vi "Copy Class.vi"(5 "Parent Class Path":path, 7 "Template Path":path, 8 "error in (no error)":errorcluster, 9 "Class Name":string, 10 "Destination Directory":path, 11 "AppInst":refnum<vi>) -> (0 "error out":errorcluster, 2 "New Class Path":path)   [LabVIEW 2020, in "Message Maker.lvlib"]
uses:
  Message Maker.lvlib
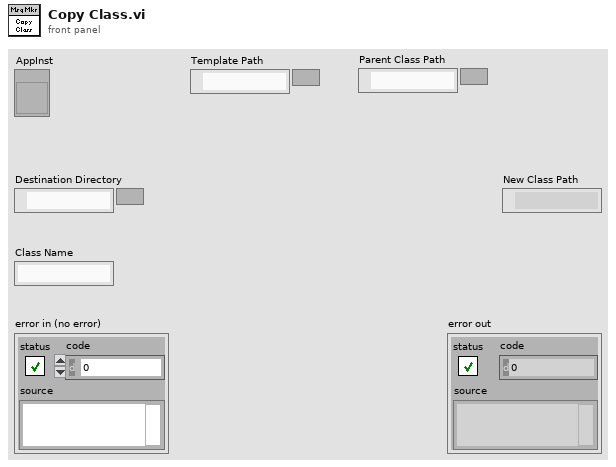
[diagram p1: front panel]
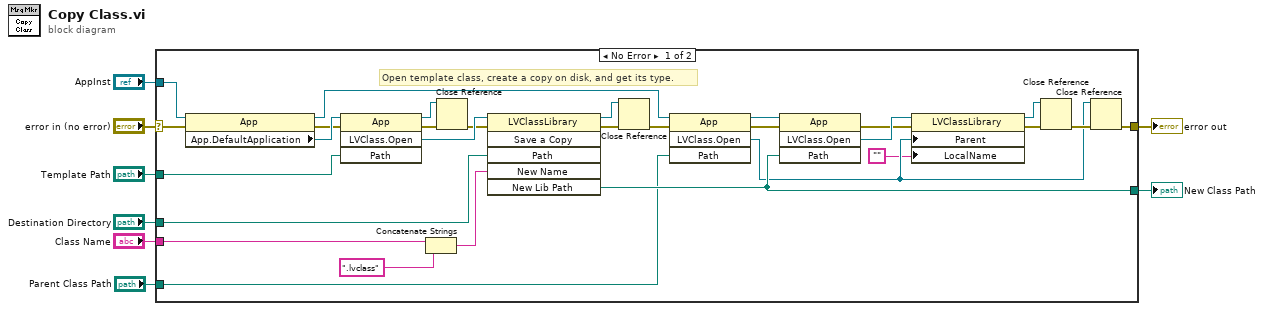
[diagram p0: block diagram]
diagram:
  n1 = case shown="No Error" "error in (no error)" {
    selector: "error in (no error)" -> [w30 w38]
    tunnel: "Template Path" -> [w29 _]
    tunnel: "Destination Directory" -> [w35 _]
    tunnel: [w26 _] -> w6
    tunnel: "Class Name" -> [w34 _]
    tunnel: [w15 w38] -> w4
    tunnel: "AppInst" -> [w12 _]
    tunnel: "Parent Class Path" -> [w10 _]
    frame No Error {
      # "Open template class, create a copy on disk, and get its type."
      n2 = property class="App"(reference=w12, error in=w30) -> (reference out=w11:refnum<vi>, error out=w27:errorcluster, "App.DefaultApplication"=w28:refnum<vi>)
      n3 = invoke class="App" method="LVClass.Open"(reference=w28, error in=w27, "Path"=w29) -> (reference out=w13:refnum<vi>, error out=w32:errorcluster, "LVClass.Open"=w37:refnum<vi>)  [unwired: 1 in, 1 out]
      n4 = Concatenate Strings(w34, ".lvclass" ("regular expression")) -> (w33:string)
      n5 = Close Reference(reference=w13, error in (no error)=w32) -> (error out=w14:errorcluster)
      n6 = invoke class="LVClassLibrary" method="Save a Copy"(reference=w37, error in=w14, "Path"=w35, "New Name"=w33) -> (reference out=w36:refnum<vi>, error out=w31:errorcluster, "New Lib Path"=w26:path)  [unwired: 2 in, 3 out]
      n7 = Close Reference(reference=w36, error in (no error)=w31) -> (error out=w24:errorcluster)
      n8 = invoke class="App" method="LVClass.Open"(reference=w11, error in=w24, "Path"=w10) -> (reference out=w22:refnum<vi>, error out=w23:errorcluster, "LVClass.Open"=w17:refnum<vi>)  [unwired: 1 in, 1 out]
      n9 = invoke class="App" method="LVClass.Open"(reference=w22, error in=w23, "Path"=w26) -> (error out=w21:errorcluster, "LVClass.Open"=w25:refnum<vi>)  [unwired: 1 in, 2 out]
      n10 = property class="LVClassLibrary"(reference=w25, error in=w21, "Parent"=w17, "LocalName"="") -> (reference out=w19:refnum<vi>, error out=w20:errorcluster)
      n11 = Close Reference(reference=w19, error in (no error)=w20) -> (error out=w18:errorcluster)
      n12 = Close Reference(reference=w17, error in (no error)=w18) -> (error out=w15:errorcluster)
    }
    frame Error {
    }
  }
  "error out" <- w4
  "New Class Path" <- w6
